vi "Exit Acq Loop.vi"(8 "error in (no error)":errorcluster, 11 "Data Cluster in":T1) -> (0 "error out":errorcluster, 3 "Data Cluster out":T1)   [LabVIEW 2018]
uses:
  controls/GLDL UI Data.ctl
  controls/Disconnect Control.ctl
  controls/Download Control.ctl
  controls/Exit Control.ctl
  controls/Date Control.ctl
  controls/IP Phone Number Control.ctl
  controls/Reboot Control.ctl
  controls/Connected Indicator.ctl
  controls/Output Indicator.ctl
  controls/Station ID Indicator.ctl
  Message Queue/All Message Queues.ctl
  Message Queue/Message Cluster.ctl
  controls/Processing Loop State.ctl
  Message Queue/GLDL Message Queue.lvlib
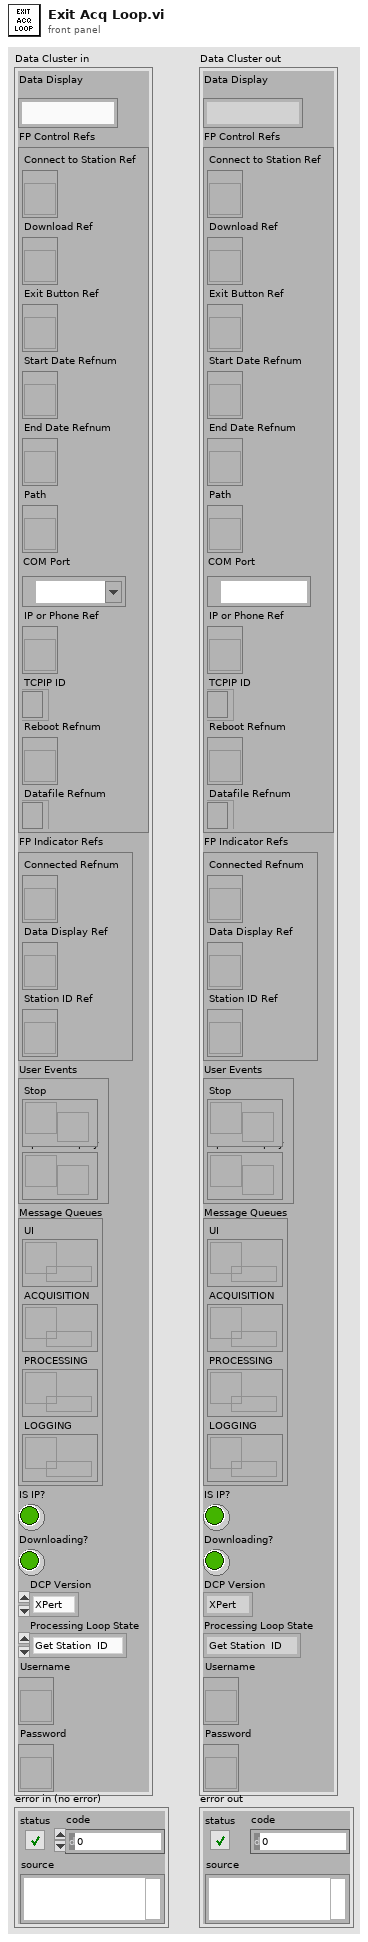
[diagram p1: front panel]
types:
  T1 = typedef "GLDL UI Data.ctl" = cluster{"Data Display":string, "FP Control Refs":cluster{"Connect to Station Ref":refnum<vi>, "Download Ref":refnum<vi>, "Exit Button Ref":refnum<vi>, "Start Date Refnum":refnum<vi>, "End Date Refnum":refnum<vi>, "Path":refnum<vi>, "COM Port":refnum<visa-resource-name>, "IP or Phone Ref":refnum<vi>, "TCPIP ID":refnum<k5>, "Reboot Refnum":refnum<vi>, "Datafile Refnum":refnum<file>}, "FP Indicator Refs":cluster{"Connected Refnum":refnum<vi>, "Data Display Ref":refnum<vi>, "Station ID Ref":refnum<vi>}, "User Events":cluster{"Stop":refnum<user-event>, "Update Display":refnum<user-event>}, "Message Queues":T2, "IS IP?":bool, "Downloading?":bool, "DCP Version":enum16{"XPert", "XPert2"}, "Processing Loop State":T3, "Username":refnum<vi>, "Password":refnum<vi>}
  T2 = typedef "GLDL Message Queue.lvlib/All Message Queues.ctl" = cluster{"UI":refnum<queue>, "ACQUISITION":refnum<queue>, "PROCESSING":refnum<queue>, "LOGGING":refnum<queue>}
  T3 = typedef "Processing Loop State.ctl" = enum16{"Get Station  ID", "Change Directory SD Card", "Change Directory Storage Card", "Downloading", "Idle in DL Directory"}
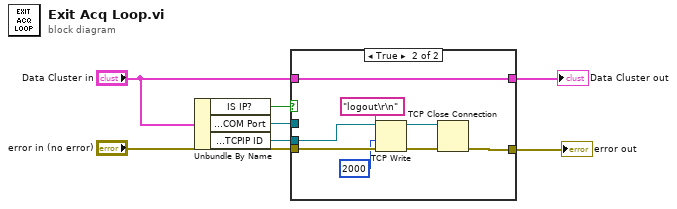
[diagram p0: block diagram]
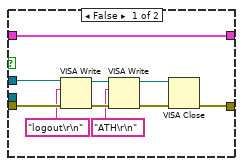
[diagram p2: hidden frame]
diagram:
  n1 = Unbundle By Name("Data Cluster in") -> ("IS IP?"=w2:bool, "FP Control Refs.COM Port"=w1:refnum<visa-resource-name>, "FP Control Refs.TCPIP ID"=w3:refnum<k5>)
  n2 = case shown="True" w2 {
    tunnel: w1 -> [w17 _]
    tunnel: w3 -> [_ w25]
    tunnel: "error in (no error)" -> [w13 w23]
    tunnel: [w14 w22] -> w5
    tunnel: "Data Cluster in" -> [w12 w18]
    tunnel: [w12 w18] -> w7
    frame False {
      n3 = VISA Write(VISA resource name=w17, write buffer="logout\r\n" ("data in"), error in (no error)=w13) -> (VISA resource name out=w11:refnum<visa-resource-name>, error out=w10:errorcluster)  [unwired: 1 out]
      n4 = VISA Write(VISA resource name=w11, write buffer="ATH\r\n" ("data in"), error in (no error)=w10) -> (VISA resource name out=w15:refnum<visa-resource-name>, error out=w16:errorcluster)  [unwired: 1 out]
      n5 = VISA Close(VISA resource name=w15, error in (no error)=w16) -> (error out=w14:errorcluster)
    }
    frame True {
      n6 = TCP Write(connection ID=w25, data in="logout\r\n", error in (no error)=w23, 9:2000 ("timeout ms (25000)")) -> (connection ID out=w20:refnum<k5>, error out=w19:errorcluster)  [unwired: 1 out]
      n7 = TCP Close Connection(connection ID=w20, error in (no error)=w19) -> (error out=w22:errorcluster)  [unwired: 1 in, 1 out]
    }
  }
  "Data Cluster out" <- w7
  "error out" <- w5
